vi "Main Page.vi"(8 "error in (no error)":errorcluster, 11 "Node Ptr":T1 format="%.0x") -> (0 "error out":errorcluster)   [LabVIEW 2015, in "Host Heartbeat System Explorer.lvlib"]
uses:
  Host Heartbeat System Explorer.lvlib
  <vilib>/NI Veristand/Custom Device API/Custom Device Item Ref.ctl
  Shared/Constants.vi
  <vilib>/NI Veristand/Custom Device API/Get Item Property (U16).vi
  <vilib>/NI Veristand/Custom Device API/Set Item Property (U16).vi
  <vilib>/NI Veristand/Custom Device API/Custom Device API.lvlib
  Shared/Host Heartbeat Shared.lvlib
panel:
  in  "Local Daemon TCP Port":u16
  in  "Target TCP Port":u16
  in  "Header":cluster{"Section Name":string}={"Section Name"="Custom Device Item Settings"}
  in  "Description":string
  in  "Name":string
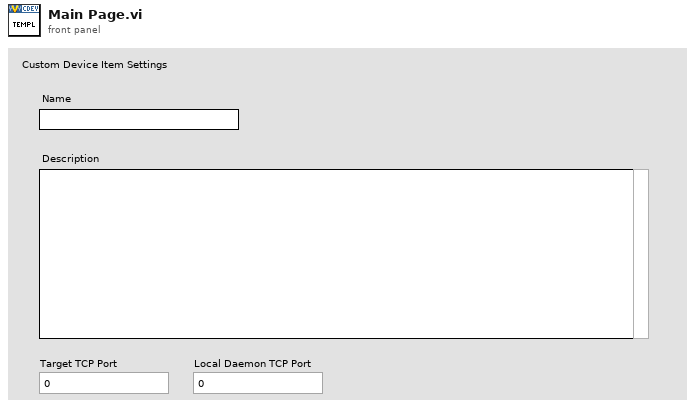
[diagram p1: front panel]
types:
  T1 = typedef "Custom Device API.lvlib/Custom Device Item Ref.ctl" = u64
  T2 = typedef "Custom Device API.lvlib/Custom Device Item Info.ctl" = cluster{"Name":string, "Is Channel":bool, "GUID":string, "Is Waveform":bool}
  T3 = typedef "Custom Device API.lvlib/Custom Device Commands.ctl" = enum16{"Default", "Item renamed", "Shutdown", "Dynamic button pressed"}
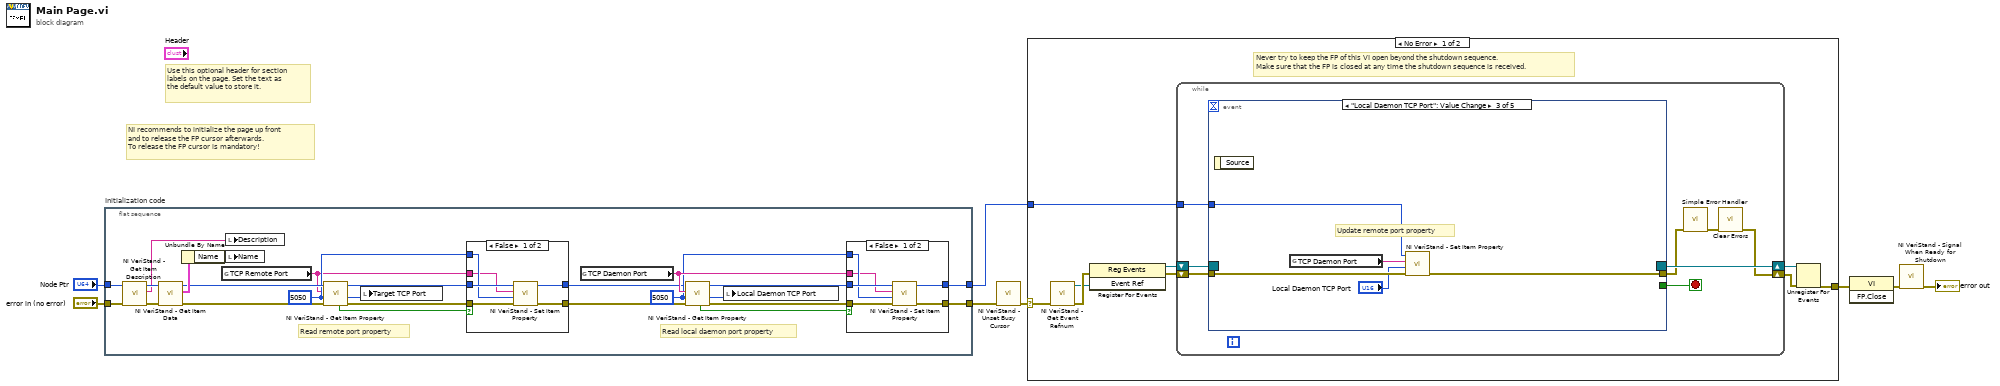
[diagram p0: block diagram]
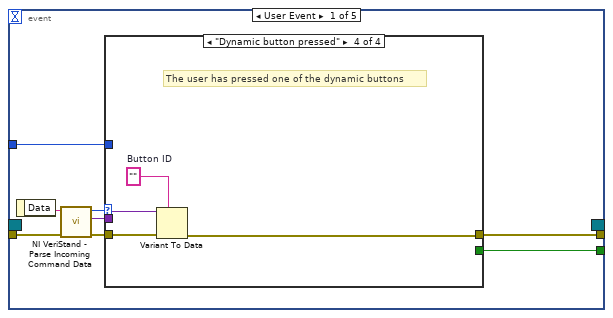
[diagram p4: hidden frame]
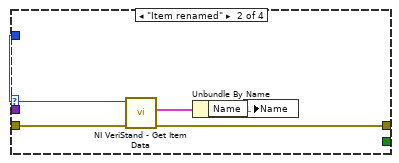
[diagram p6: hidden frame]
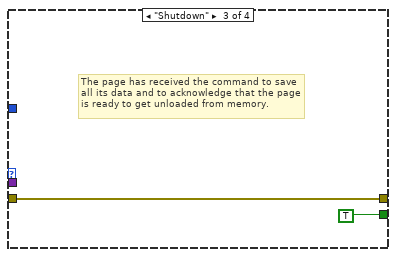
[diagram p7: hidden frame]
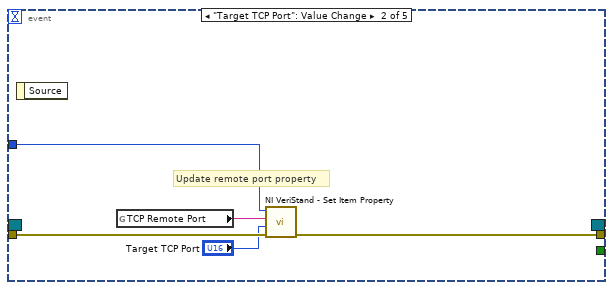
[diagram p8: hidden frame]
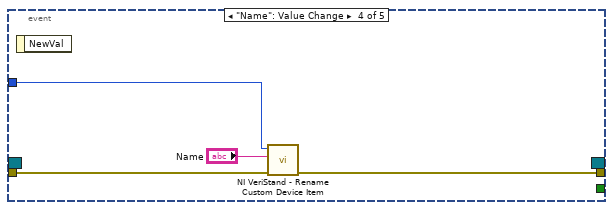
[diagram p9: hidden frame]
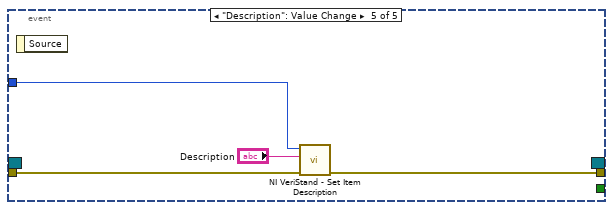
[diagram p10: hidden frame]
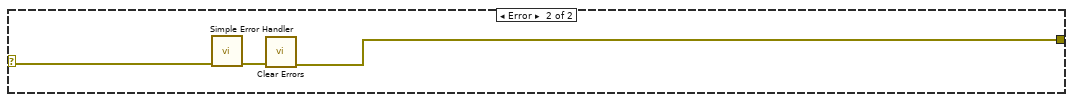
[diagram p11: hidden frame]
diagram:
  # "Use this optional header for section labels on the page. Set the text as the default value to store it."
  # "NI recommends to initialize the page up front\nand to release the FP cursor afterwards.\nTo release the FP cursor is mandatory!"
  n1 = flat-sequence "Initialization code" {
    tunnel: "error in (no error)" -> [w32]
    tunnel: "Node Ptr" -> [w31]
    tunnel: [w9] -> w4
    tunnel: [w10] -> w1
    frame #0 {
      w17 = u16 5050 ("Default Value")
      w20 = u16 5050 ("Default Value")
      # "Read local daemon port property"
      # "Read remote port property"
      n2 = call <vilib>:"NI VeriStand - Get Item Description.vi"("error in (no error)"=w32, "Item Ref in"=w31) -> ("error out"=w29:errorcluster, "Description"=w30:string, "Item Ref out"=w33:T1)  [unwired: 7 out]
      n3 = call <vilib>:"NI VeriStand - Get Item Data.vi"("error in (no error)"=w29, "Item Ref in"=w33) -> ("error out"=w26:errorcluster, "Item Info"=w28:T2, "Item Ref out"=w25:T1)  [unwired: 7 out]
      n4 = Unbundle By Name(w28) -> ("Name"=w27:string)
      n5 = global read "Constants.vi" "TCP Remote Port"() -> (w19:string)
      n6 = local write "Description"(w30) -> ()
      n7 = local write "Name"(w27) -> ()
      n8 = call-poly <vilib>:"NI VeriStand - Get Item Property.vi"("error in (no error)"=w26, "Default Value"=w20, "Property Name"=w19, "Item Ref in"=w25) -> ("error out"=w21:errorcluster, "Value"=w24:u16, "Item Ref out"=w22:T1, "Found?"=w23:bool)  [unwired: 4 in]
      n9 = local write "Target TCP Port"(w24) -> ()
      n10 = case shown="False" w23 {
        tunnel: w22 -> [w47 w48]
        tunnel: w21 -> [w44 w49]
        tunnel: [w43 w49] -> w11
        tunnel: [w42 w48] -> w12
        tunnel: w20 -> [w46 _]
        tunnel: w19 -> [w45 _]
        frame False {
          n11 = call-poly <vilib>:"NI VeriStand - Set Item Property.vi"("error in (no error)"=w44, "Value"=w46, "Property Name"=w45, "Item Ref in"=w47) -> ("error out"=w43:errorcluster, "Item Ref out"=w42:T1)  [unwired: 5 in, 1 out]
        }
        frame True {
        }
      }
      n12 = global read "Constants.vi" "TCP Daemon Port"() -> (w18:string)
      n13 = call-poly <vilib>:"NI VeriStand - Get Item Property.vi"("error in (no error)"=w11, "Default Value"=w17, "Property Name"=w18, "Item Ref in"=w12) -> ("error out"=w16:errorcluster, "Value"=w13:u16, "Item Ref out"=w15:T1, "Found?"=w14:bool)  [unwired: 4 in]
      n14 = local write "Local Daemon TCP Port"(w13) -> ()
      n15 = case shown="False" w14 {
        tunnel: w15 -> [w39 w40]
        tunnel: w16 -> [w36 w41]
        tunnel: [w35 w41] -> w9
        tunnel: [w34 w40] -> w10
        tunnel: w17 -> [w38 _]
        tunnel: w18 -> [w37 _]
        frame False {
          n16 = call-poly <vilib>:"NI VeriStand - Set Item Property.vi"("error in (no error)"=w36, "Value"=w38, "Property Name"=w37, "Item Ref in"=w39) -> ("error out"=w35:errorcluster, "Item Ref out"=w34:T1)  [unwired: 5 in, 1 out]
        }
        frame True {
        }
      }
    }
  }
  n17 = call <vilib>:"NI VeriStand - Unset Busy Cursor.vi"("error in (no error)"=w4) -> ("error out"=w3:errorcluster)  [unwired: 10 out]
  n18 = case shown="No Error" w3 {
    selector: w3 -> [w50 w107]
    tunnel: [w55 w105] -> w8
    tunnel: w1 -> [w51 _]
    frame No Error {
      # "Never try to keep the FP of this VI open beyond the shutdown sequence.\nMake sure that the FP is closed at any time the shutdown sequence is received."
      n19 = call <vilib>:"NI VeriStand - Get Event Refnum.vi"("error in (no error)"=w50) -> ("error out"=w58:errorcluster, "Event Ref"=w54:refnum<user-event>)  [unwired: 9 out]
      n20 = register-events(error in=w58, w54) -> (reference out=w52:refnum<event-registration>, error out=w53:errorcluster)  [unwired: 1 in]
      n21 = while {
        tunnel: w51 -> [w62]
        shift-right: [w59] -> w56
        shift-left: w53 -> [w65]
        shift-right: [w66] -> w57
        shift-left: w52 -> [w64]
        stop <- w63 stop-if-true
        n22 = event shown="[2] \"Local Daemon TCP Port\": Value Change" {
          selector: w64 -> [_ _ _ _ _]
          dyn-events: [_ _ _ _ _] -> w66
          timeout: _ -> [_ _ _ _ _]
          tunnel: w65 -> [w74 w90 w95 w100 w103]
          tunnel: [w70 _ _ _ _] -> w63
          tunnel: [w69 w89 w94 w99 w102] -> w61
          tunnel: w62 -> [w68 w91 w96 w98 w104]
          event User Event {
            n23 = event-data() -> ("Data"=w73:string)  [unwired: 1 out]
            n24 = call <vilib>:"NI VeriStand - Parse Incoming Command Data.vi"("error in (no error)"=w74, "Incoming data"=w73) -> ("error out"=w72:errorcluster, "Outgoing data"=w67:variant, "Action"=w71:T3)  [unwired: 7 out]
            n25 = case shown="\"Dynamic button pressed\"" w71 {
              tunnel: w72 -> [w75 w80 w81 w86]
              tunnel: [_ _ TRUE _] -> w70
              tunnel: [w75 w77 w81 w83] -> w69
              tunnel: w68 -> [_ w79 _ _]
              tunnel: w67 -> [_ _ _ w85]
              frame "Default", Default {
              }
              frame "Item renamed" {
                n26 = call <vilib>:"NI VeriStand - Get Item Data.vi"("error in (no error)"=w80, "Item Ref in"=w79) -> ("error out"=w77:errorcluster, "Item Info"=w78:T2)  [unwired: 8 out]
                n27 = Unbundle By Name(w78) -> ("Name"=w76:string)
                n28 = local write "Name"(w76) -> ()
              }
              frame "Shutdown" {
                # "The page has received the command to save all its data and to acknowledge that the page is ready to get unloaded from memory."
              }
              frame "Dynamic button pressed" {
                w84 = ""  # Button ID
                # "The user has pressed one of the dynamic buttons"
                n29 = Variant To Data(error in=w86, type=w84, Variant=w85) -> (error out=w83:errorcluster)  [unwired: 1 out]
              }
            }
          }
          event "Target TCP Port": Value Change {
            # "Update remote port property"
            n30 = event-data() -> ()  [unwired: 2 out]
            n31 = global read "Constants.vi" "TCP Remote Port"() -> (w88:string)
            n32 = call-poly <vilib>:"NI VeriStand - Set Item Property.vi"("error in (no error)"=w90, "Value"="Target TCP Port", "Property Name"=w88, "Item Ref in"=w91) -> ("error out"=w89:errorcluster)  [unwired: 5 in, 2 out]
          }
          event "Local Daemon TCP Port": Value Change {
            # "Update remote port property"
            n33 = event-data() -> ()  [unwired: 2 out]
            n34 = global read "Constants.vi" "TCP Daemon Port"() -> (w93:string)
            n35 = call-poly <vilib>:"NI VeriStand - Set Item Property.vi"("error in (no error)"=w95, "Value"="Local Daemon TCP Port", "Property Name"=w93, "Item Ref in"=w96) -> ("error out"=w94:errorcluster)  [unwired: 5 in, 2 out]
          }
          event "Name": Value Change {
            n36 = event-data() -> ()  [unwired: 2 out]
            n37 = call <vilib>:"NI VeriStand - Rename Custom Device Item.vi"("error in (no error)"=w100, "New Name"="Name", "Item Ref in"=w98) -> ("error out"=w99:errorcluster)  [unwired: 1 in, 7 out]
          }
          event "Description": Value Change {
            n38 = event-data() -> ()  [unwired: 2 out]
            n39 = call <vilib>:"NI VeriStand - Set Item Description.vi"("error in (no error)"=w103, "Description"="Description", "Item Ref in"=w104) -> ("error out"=w102:errorcluster)  [unwired: 8 out]
          }
        }
        n40 = call <vilib>:"Simple Error Handler.vi"("error in (no error)"=w61) -> ("error out"=w60:errorcluster)  [unwired: 1 in, 7 out]
        n41 = call <vilib>:"Clear Errors.vi"("error in (no error)"=w60) -> ("error out"=w59:errorcluster)  [unwired: 1 in, 5 out]
      }
      n42 = Unregister For Events(event registration refnum=w57, error in=w56) -> (error out=w55:errorcluster)
    }
    frame Error {
      n43 = call <vilib>:"Simple Error Handler.vi"("error in (no error)"=w107) -> ("error out"=w106:errorcluster)  [unwired: 1 in, 7 out]
      n44 = call <vilib>:"Clear Errors.vi"("error in (no error)"=w106) -> ("error out"=w105:errorcluster)  [unwired: 1 in, 5 out]
    }
  }
  n45 = invoke class="VI" method="FP.Close"(error in=w8) -> (error out=w7:errorcluster)  [unwired: 2 in, 2 out]
  n46 = call <vilib>:"NI VeriStand - Signal When Ready for Shutdown.vi"("error in (no error)"=w7) -> ("error out"=→"error out":errorcluster)  [unwired: 10 out]
